vi "MultiChannel Write.vi"(8 "Error In":errorcluster, 10 "Data to Log":dbl[][](array[numeric]), 11 "File Refnum In":refnum<file>) -> (0 "Error Out":errorcluster, 3 "File Refnum Out":refnum<file>)   [LabVIEW 2014]
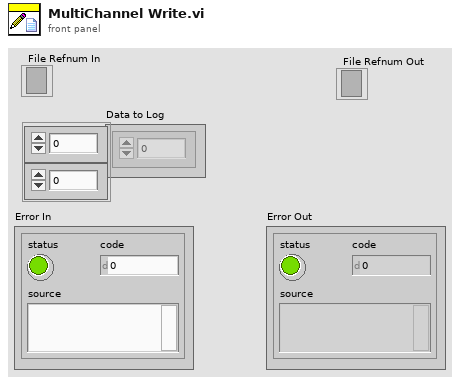
[diagram p1: front panel]
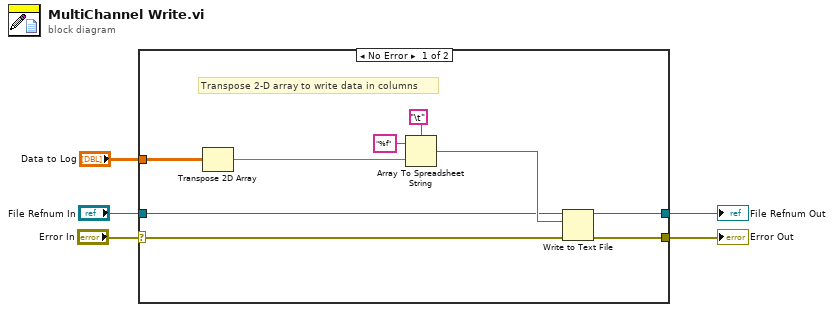
[diagram p0: block diagram]
diagram:
  n1 = case shown="No Error" "Error In" {
    selector: "Error In" -> [w14 w16]
    tunnel: "File Refnum In" -> [w7 w15]
    tunnel: [w6 w15] -> w3
    tunnel: [w13 w16] -> w2
    tunnel: "Data to Log" -> [w9 _]
    frame No Error {
      # "Transpose 2-D array to write data in columns"
      n2 = Transpose 2D Array(2D array=w9) -> (transposed array=w8:dbl[][])
      n3 = Array To Spreadsheet String(delimiter (Tab)="\t", array=w8, 3:"%f" ("format string")) -> (spreadsheet string=w12:string)
      n4 = Write to Text File(file (use dialog)=w7, text=w12, error in=w14) -> (refnum out=w6:refnum<file>, error out=w13:errorcluster)  [unwired: 1 in, 1 out]
    }
    frame Error {
    }
  }
  "Error Out" <- w2
  "File Refnum Out" <- w3
